vi "ReadB.vi"(1 "Offset":u32) -> (0 "Data":u8=255)   [LabVIEW 2015]
uses:
  lv64_eventdriven2015/board.vis/ESLSCDLL.dll
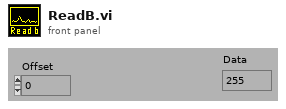
[diagram p1: front panel]
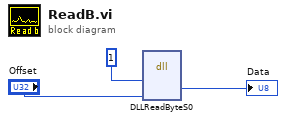
[diagram p0: block diagram]
diagram:
  n1 = dll-call lib="C:/ENTW/PCIE/64bit/lv64/lv64_eventdriven2015/board.vis/ESLSCDLL.dll" fn="DLLReadByteS0"("drv"=u32 1, "PortOff"="Offset") -> ("data"=→"Data":u8)  [unwired: 7 in, 2 out]
